vi "Update charts.vi"(8 "error in (no error)":errorcluster, 11 "Main UI in":refnum<class "Main UI.lvclass">) -> (0 "error out":errorcluster, 3 "Main UI out":refnum<class "Main UI.lvclass">)   [LabVIEW 2011, in "Main UI.lvclass"]
uses:
  Main UI.lvclass
  Main UI.lvclass/Main UI.ctl
panel:
  in  "Cluster":cluster{"EDR":dbl, "Pulse":dbl}
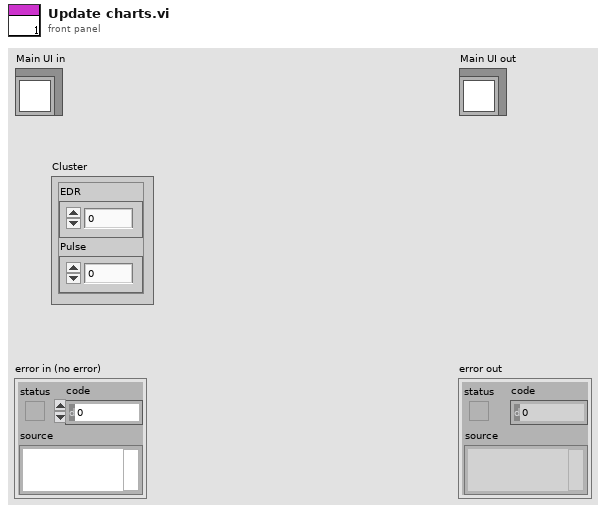
[diagram p1: front panel]
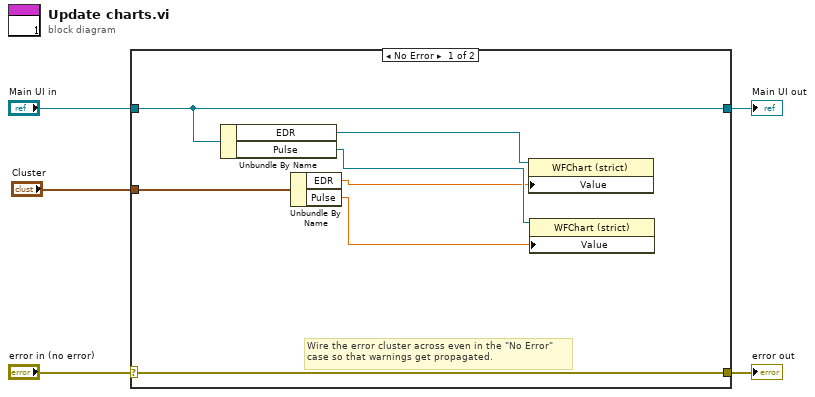
[diagram p0: block diagram]
diagram:
  n1 = case shown="No Error" "error in (no error)" {
    selector: "error in (no error)" -> [w12 w14]
    tunnel: [w12 w14] -> w4
    tunnel: [w11 w13] -> w2
    tunnel: "Main UI in" -> [w11 w13]
    tunnel: "Cluster" -> [w10 _]
    frame No Error {
      # "Wire the error cluster across even in the \"No Error\"\ncase so that warnings get propagated."
      n2 = Unbundle By Name(w11) -> ("EDR"=w9:refnum<vi>, "Pulse"=w8:refnum<vi>)
      n3 = Unbundle By Name(w10) -> ("EDR"=w7:dbl, "Pulse"=w6:dbl)
      n4 = property class="WFChart (strict)"(reference=w9, "Value"=w7) -> ()  [unwired: 1 in, 2 out]
      n5 = property class="WFChart (strict)"(reference=w8, "Value"=w6) -> ()  [unwired: 1 in, 2 out]
    }
    frame Error {
    }
  }
  "error out" <- w4
  "Main UI out" <- w2
